vi "Cleanup.vi"(8 "error in (no error)":errorcluster, 11 "WebProjectPanel in":refnum<class "WebProjectPanel.lvclass">) -> (0 "error out":errorcluster)   [LabVIEW 2020, in "PicoG-Processor.lvlib" / "WebProjectPanel.lvclass"]
uses:
  WebProjectPanel.lvclass
  WebProjectPanel.lvclass/WebProjectPanel.ctl
  <vilib>/IlluminatedG/IG OOPanel/OOPanel/ArrayPanel/ArrayPanel.lvclass
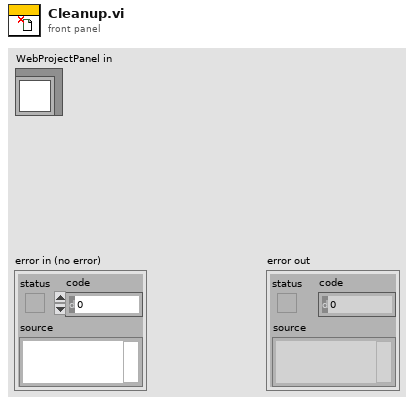
[diagram p1: front panel]
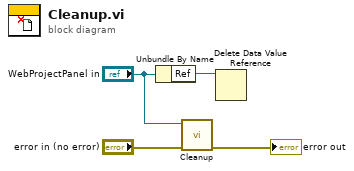
[diagram p0: block diagram]
diagram:
  n1 = Unbundle By Name("WebProjectPanel in") -> ("Ref"=w3:refnum<data-value>)
  n2 = call-parent "Cleanup.vi"("error in (no error)"="error in (no error)", "ArrayPanel in"="WebProjectPanel in") -> ("error out"=→"error out":errorcluster)  [unwired: 9 in]
  n3 = Delete Data Value Reference(data value reference=w3) -> ()  [unwired: 1 in, 2 out]
